vi "MatrixB.vi"(0 "No record Vg rate (V/min)":dbl=150.0, 3 "Time Stamp":timestamp, 4 "Voltage (sourse)":dbl, 6 "Play Button":bool, 8 "Custom Folder":string, 9 "Settings":T1={"Ring 3"=1, "Ring 2"=4, "Fixed Current mkA"=0.5, "If yes, the current is:"=enum."Radio Selection 1", "Ressitance measurements?"=TRUE, "Commute DC current?"=FALSE} {"Ring 3" items=["1 kOhm", "10 kOhm", "100 kOhm", "1 Mohm", "10 mOhm"]; "Ring 2" items=["1 kOhm", "10 kOhm", "100 kOhm", "1 Mohm", "10 MOhm"]}, 10 "Instruments":T2={"Oscillator"=TRUE, "Addr 1 lock-in"=TRUE, "Addr 1 lock-in oop"=TRUE, "Addr 2 lock-in"=TRUE, "Addr 2 lock-in oop"=TRUE, "Addr 3 lock-in"=FALSE, "Addr 3 lock-in oop"=FALSE, "Voltage (Vk1)"=TRUE, "Current (Ik1)"=TRUE, "Voltage (Vk2)"=FALSE, "Current (Ik2)"=FALSE, "Voltage (Vk3)"=FALSE, "Current (Ik3)"=FALSE, "Channel 1 (Vnano1)  "=FALSE, "Channel 2 (Vnano1b)"=FALSE, "Channel 1 (Vnano2)   "=FALSE, "Channel 2 (Vnano2b)"=FALSE, "Thermometer 1 (T1)"=TRUE, "Magnetic Field (B)"=TRUE, "Capacitance (C) and Loss (L)"=FALSE}, 11 "BCluster":T3={"B1 (T)"=-1.0, "B2 (T)"=1.0, "Sweep rate, T/min"=0.5, "Time btw \npoints, sec"=1.0, "No-record rate, T/min"=0.5, "Full sweep?"=FALSE, "Odd confgurations"=TRUE} {"No-record rate, T/min" min=0.0 max=1.0 step=0.01 format="%_4f"; "B2 (T)" min=-4.0 max=4.0 step=0.1 format="%.1f"; "Time btw \npoints, sec" format="%.2f"; "Sweep rate, T/min" min=0.0 max=1.0 step=0.01 format="%_4f"; "B1 (T)" min=-4.0 max=4.0 step=0.1 format="%.1f"}) -> ()   [LabVIEW 2017]
uses:
  <vilib>/Utility/file.llb/Read From Spreadsheet File (DBL).vi
panel:
  out "ArraySens 2":i8[](array[numeric])
  out "String":string
  out "Experiment ends at:":string
  out "Hours":dbl format="%.1f"
  out "Estimated time of experiment:":i16
  out "ArraySens":i8[](array[numeric])
  out "ArrayOsc":dbl[](array[numeric])
  out "# of configurations":i8
  out "Large Array":bool[][][](array[boolean])
  out "Contact configuration file (*.conf)":path
  # "hours"
  # "min.="
  # "Lock-in Amplifiers"
  # "Temperature"
  # "SourceMeters"
  # "Nanovoltmeters"
  # "Main"
  # "(not recommended, too slow)"
  # "Magnetic Field"
  # "Capacitance & Loss"
  # "(not recommended, too slow)"
  # ": B1 to B2, even: B2 to B1"
  # "(For hysteresis measurements)"
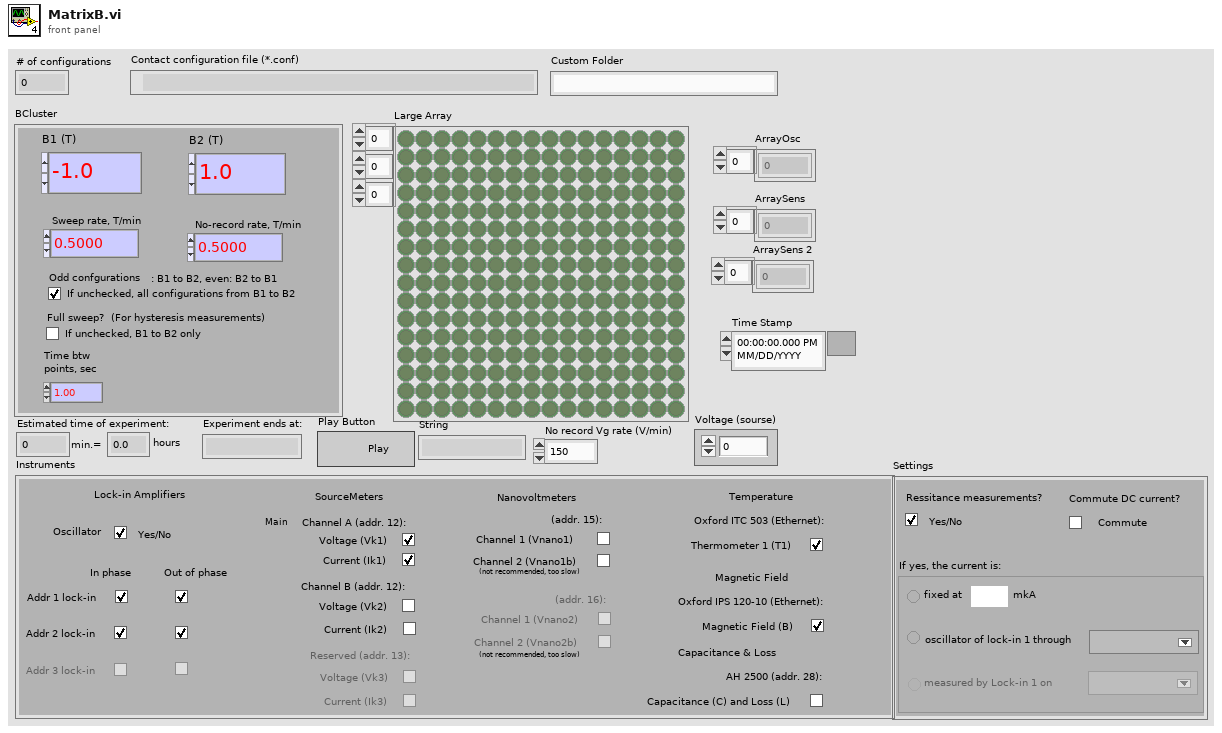
[diagram p1: front panel]
types:
  T1 = cluster{"Ring 3":u16, "Ring 2":u16, "Fixed Current mkA":dbl, "If yes, the current is:":enum32{"Radio Selection 1", "Radio Selection 2", "Radio Selection 3"}, "Ressitance measurements?":bool, "Commute DC current?":bool}
  T2 = cluster{"Oscillator":bool, "Addr 1 lock-in":bool, "Addr 1 lock-in oop":bool, "Addr 2 lock-in":bool, "Addr 2 lock-in oop":bool, "Addr 3 lock-in":bool, "Addr 3 lock-in oop":bool, "Voltage (Vk1)":bool, "Current (Ik1)":bool, "Voltage (Vk2)":bool, "Current (Ik2)":bool, "Voltage (Vk3)":bool, "Current (Ik3)":bool, "Channel 1 (Vnano1)  ":bool, "Channel 2 (Vnano1b)":bool, "Channel 1 (Vnano2)   ":bool, "Channel 2 (Vnano2b)":bool, "Thermometer 1 (T1)":bool, "Magnetic Field (B)":bool, "Capacitance (C) and Loss (L)":bool}
  T3 = cluster{"B1 (T)":dbl, "B2 (T)":dbl, "Sweep rate, T/min":dbl, "Time btw \npoints, sec":dbl, "No-record rate, T/min":dbl, "Full sweep?":bool, "Odd confgurations":bool}
  T4 = cluster{"B1 (T)":dbl, "Sweep rate, T/min":dbl, "Time btw \npoints, sec":dbl}
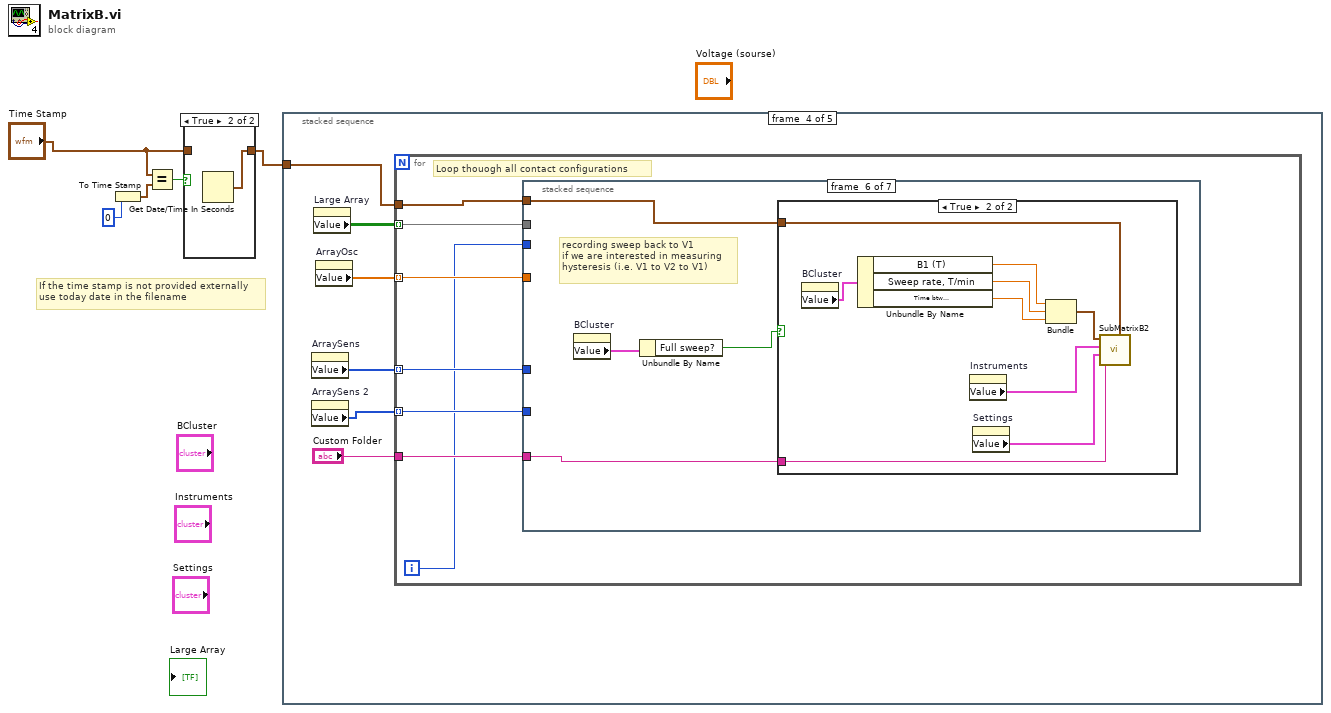
[diagram p0: block diagram]
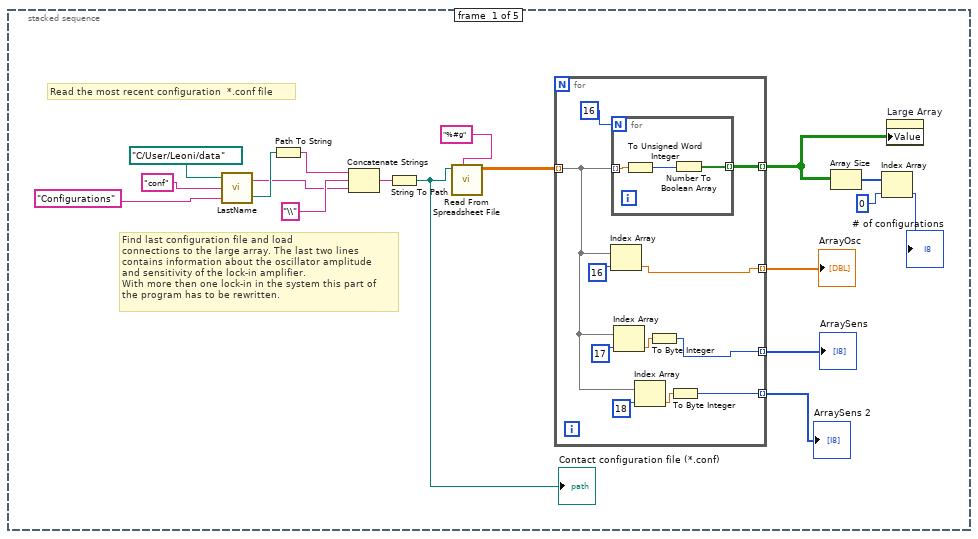
[diagram p3: hidden frame]
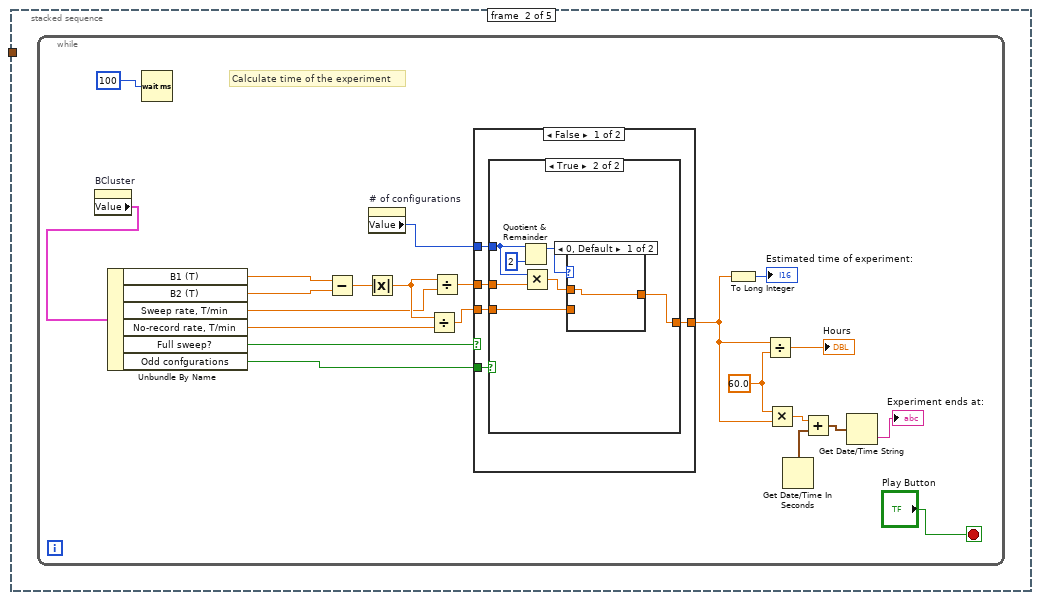
[diagram p4: hidden frame]
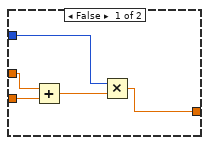
[diagram p5: hidden frame]
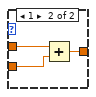
[diagram p6: hidden frame]
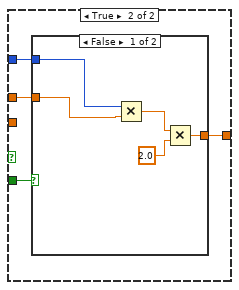
[diagram p7: hidden frame]
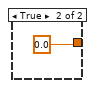
[diagram p8: hidden frame]
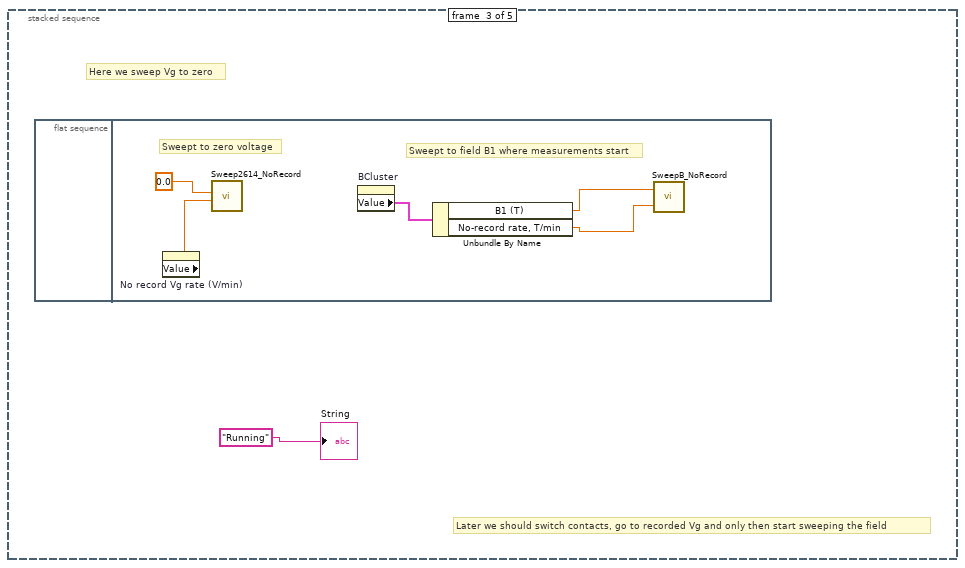
[diagram p9: hidden frame]
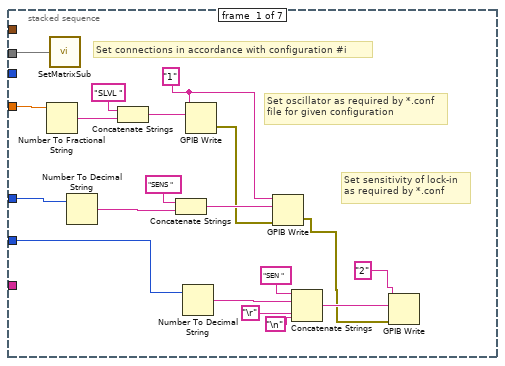
[diagram p10: hidden frame]
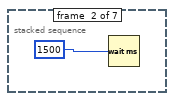
[diagram p11: hidden frame]
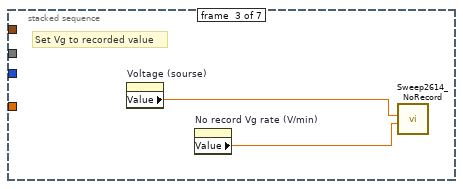
[diagram p12: hidden frame]
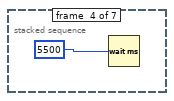
[diagram p13: hidden frame]
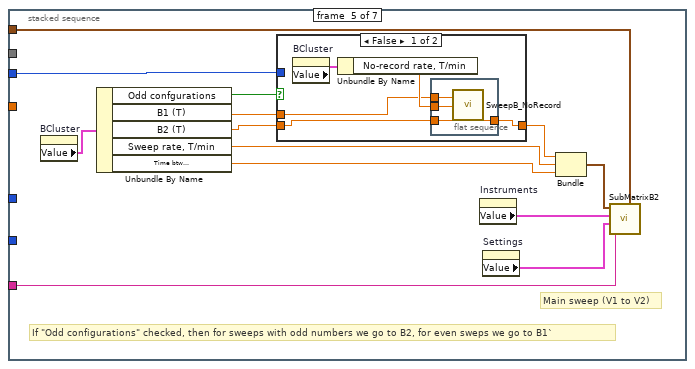
[diagram p14: hidden frame]
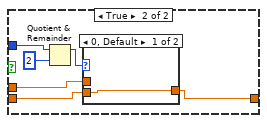
[diagram p15: hidden frame]
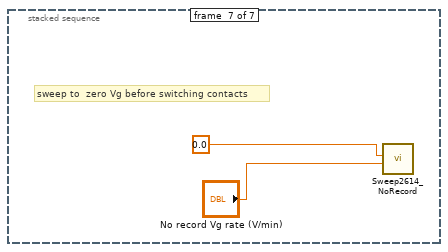
[diagram p18: hidden frame]
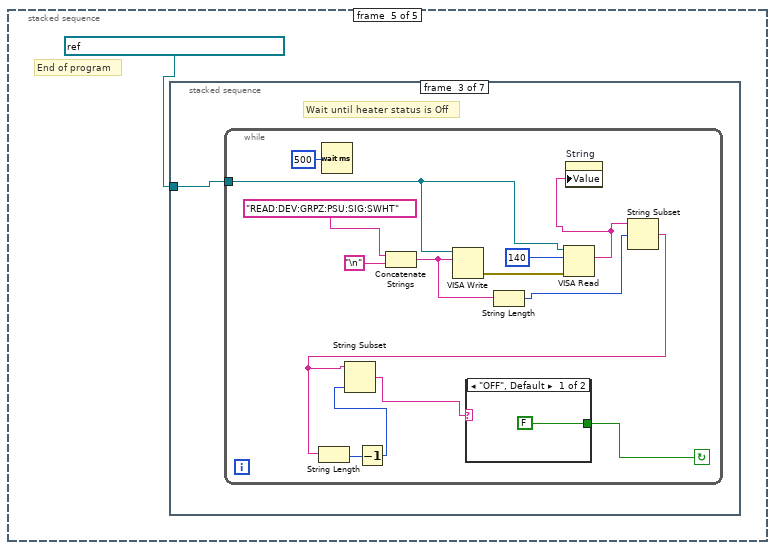
[diagram p19: hidden frame]
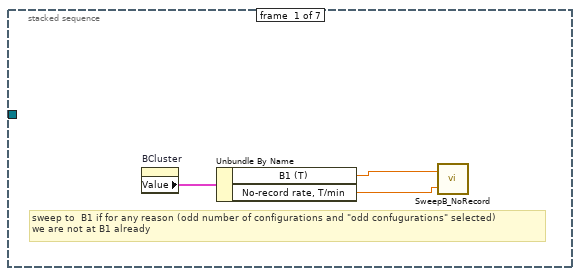
[diagram p20: hidden frame]
diagram:
  # "If the time stamp is not provided externally\nuse today date in the filename"
  n1 = To Time Stamp(1:0) -> (0:w4:timestamp)
  n2 = Equal?(x="Time Stamp", y=w4) -> (x = y?=w3:bool)
  n3 = case shown="True" w3 {
    tunnel: "Time Stamp" -> [w6 _]
    tunnel: [w6 w7] -> w1
    frame False {
    }
    frame True {
      n4 = Get Date/Time In Seconds() -> (seconds since 1Jan1904=w7:timestamp)
    }
  }
  n5 = stacked-sequence {
    tunnel: w1 -> [_ _ _ w100 _]
    frame #0 {
      # "Read the most recent configuration  *.conf file"
      # "Find last configuration file and load \nconnections to the large array. The last two lines \ncontains information about the oscillator amplitude\nand sensitivity of the lock-in amplifier.\nWith more then one lock-in in the system this part of \nthe program has to be rewritten."
      n6 = call "LastName.vi"("Custom Folder"="Configurations", "Extention"="conf", "User Data Folder"=path "C:/User/Leoni/data") -> ("created path"=w21:path, "String"=w20:string)
      n7 = Path To String(path=w21) -> (string=w25:string)
      n8 = Concatenate Strings(w25, "\\", w20) -> (w23:string)
      n9 = String To Path(string=w23) -> (path=w11:path)
      "Contact configuration file (*.conf)" <- w11
      n10 = call-poly <vilib>:"Read From Spreadsheet File.vi"("format (%.3f)"="%#g", "file path (dialog if empty)"=w11) -> ("all rows"=w16:dbl[][])  [unwired: 5 in, 4 out]
      n11 = for {
        tunnel: w16 -> [w27] mode=indexing
        tunnel: [w36] -> w13 mode=indexing
        tunnel: [w32] -> w10 mode=indexing
        tunnel: [w31] -> w9 mode=indexing
        tunnel: [w26] -> w8 mode=indexing
        n12 = Index Array(array=w27, index=16) -> (element=w32:dbl)
        n13 = for {
          N: 16 -> [_]
          tunnel: w27 -> [w39] mode=indexing
          tunnel: [w37] -> w36 mode=indexing
          n14 = To Unsigned Word Integer(number=w39) -> (unsigned 16bit integer=w38:u16)
          n15 = Number To Boolean Array(number=w38) -> (Boolean array=w37:bool[])
        }
        n16 = Index Array(array=w27, index=17) -> (element=w33:dbl)
        n17 = Index Array(array=w27, index=18) -> (element=w28:dbl)
        n18 = To Byte Integer(number=w33) -> (8bit integer=w31:i8)
        n19 = To Byte Integer(number=w28) -> (8bit integer=w26:i8)
      }
      "ArrayOsc" <- w10
      "ArraySens" <- w9
      "ArraySens 2" <- w8
      n20 = Array Size(array=w13) -> (size(s)=w15:i32[])
      n21 = Index Array(array=w15, index=0) -> (element=→"# of configurations":i32)
      n22 = property on="Large Array" class="Arr (strict)"("Value"=w13) -> ()  [unwired: 2 in, 2 out]
    }
    frame #1 {
      n23 = while {
        stop <- "Play Button" stop-if-true
        w47 = 60.0
        # "Calculate time of the experiment"
        n24 = property on="BCluster" class="Clust (strict)"() -> ("Value"=w59:T3)  [unwired: 2 in, 2 out]
        n25 = Unbundle By Name(w59) -> ("B1 (T)"=w58:dbl, "B2 (T)"=w57:dbl, "Sweep rate, T/min"=w54:dbl, "No-record rate, T/min"=w53:dbl, "Full sweep?"=w42:bool, "Odd confgurations"=w41:bool)
        n26 = Wait (ms)(milliseconds to wait=100) -> ()  [unwired: 1 out]
        n27 = Subtract(x=w58, y=w57) -> (x-y=w56:dbl)
        n28 = Absolute Value(x=w56) -> (abs(x)=w55:dbl)
        n29 = property on="# of configurations" class="DigNum (strict)"() -> ("Value"=w40:i8)  [unwired: 2 in, 2 out]
        n30 = Divide(x=w55, y=w53) -> (x/y=w43:dbl)
        n31 = Divide(x=w55, y=w54) -> (x/y=w44:dbl)
        n32 = case shown="False" w42 {
          tunnel: [w62 w86] -> w46
          tunnel: w44 -> [w66 w84]
          tunnel: w43 -> [w65 _]
          tunnel: w40 -> [w64 w83]
          tunnel: w41 -> [w63 w85]
          frame False {
            n33 = case shown="True" w63 {
              tunnel: w66 -> [w71 w75]
              tunnel: w65 -> [w70 w73]
              tunnel: w64 -> [w68 w76]
              tunnel: [w67 w72] -> w62
              frame False {
                n34 = Add(x=w71, y=w70) -> (x+y=w69:dbl)
                n35 = Multiply(x=w68, y=w69) -> (x*y=w67:dbl)
              }
              frame True {
                n36 = Quotient & Remainder(x=w76, y=2) -> (x-y*floor(x/y)=w77:i32)  [unwired: 1 out]
                n37 = Multiply(x=w76, y=w75) -> (x*y=w74:dbl)
                n38 = case shown="0, Default" w77 {
                  tunnel: w74 -> [w79 w82]
                  tunnel: w73 -> [_ w81]
                  tunnel: [w79 w80] -> w72
                  frame 0, Default {
                  }
                  frame 1 {
                    n39 = Add(x=w82, y=w81) -> (x+y=w80:dbl)
                  }
                }
              }
            }
          }
          frame True {
            n40 = case shown="False" w85 {
              tunnel: [w90 0.0] -> w86
              tunnel: w84 -> [w89 _]
              tunnel: w83 -> [w88 _]
              frame False {
                n41 = Multiply(x=w88, y=w89) -> (x*y=w87:dbl)
                n42 = Multiply(x=w87, y=2.0) -> (x*y=w90:dbl)
              }
              frame True {
              }
            }
          }
        }
        n43 = To Long Integer(number=w46) -> (32bit integer=→"Estimated time of experiment:":i32)
        n44 = Divide(x=w46, y=w47) -> (x/y=→"Hours":dbl)
        n45 = Multiply(x=w47, y=w46) -> (x*y=w45:dbl)
        n46 = Get Date/Time In Seconds() -> (seconds since 1Jan1904=w51:timestamp)
        n47 = Add(x=w45, y=w51) -> (x+y=w50:timestamp)
        n48 = Get Date/Time String(seconds (now)=w50) -> (time string=→"Experiment ends at:":string)  [unwired: 2 in, 1 out]
      }
    }
    frame #2 {
      # "Later we should switch contacts, go to recorded Vg and only then start sweeping the field"
      # "Here we sweep Vg to zero"
      n49 = flat-sequence {
        frame #0 {
        }
        frame #1 {
          # "Sweept to field B1 where measurements start"
          # "Sweept to zero voltage"
          n50 = property on="No record Vg rate (V/min)" class="DigNum (strict)"() -> ("Value"=w98:dbl)  [unwired: 2 in, 2 out]
          n51 = call "Sweep2614_NoRecord.vi"("Rate (V/min)"=w98, "Vfinal (V)"=0.0) -> ()  [unwired: 2 in, 1 out]
          n52 = property on="BCluster" class="Clust (strict)"() -> ("Value"=w96:T3)  [unwired: 2 in, 2 out]
          n53 = Unbundle By Name(w96) -> ("B1 (T)"=w94:dbl, "No-record rate, T/min"=w95:dbl)
          n54 = call "SweepB_NoRecord.vi"("Sweep Rate w/o recording (T/min)"=w95, "Target Field (T)"=w94) -> ()  [unwired: 2 in]
        }
      }
      "String" <- "Running"
    }
    frame #3 {
      n55 = property on="ArraySens" class="Arr (strict)"() -> ("Value"=w102:i8[])  [unwired: 2 in, 2 out]
      n56 = property on="ArraySens 2" class="Arr (strict)"() -> ("Value"=w99:i8[])  [unwired: 2 in, 2 out]
      n57 = property on="Large Array" class="Arr (strict)"() -> ("Value"=w104:bool[][][])  [unwired: 2 in, 2 out]
      n58 = property on="ArrayOsc" class="Arr (strict)"() -> ("Value"=w103:dbl[])  [unwired: 2 in, 2 out]
      n59 = for {
        tunnel: w104 -> [w111] mode=indexing
        tunnel: w103 -> [w110] mode=indexing
        tunnel: w102 -> [w109] mode=indexing
        tunnel: "Custom Folder" -> [w108]
        tunnel: w100 -> [w107]
        tunnel: w99 -> [w106] mode=indexing
        i -> [w105]
        # "Loop thouogh all contact configurations"
        n60 = stacked-sequence {
          tunnel: w111 -> [w130 _ _ _ _ _ _]
          tunnel: w110 -> [w126 _ _ _ _ _ _]
          tunnel: w109 -> [w121 _ _ _ _ _ _]
          tunnel: w108 -> [_ _ _ _ w147 w167 _]
          tunnel: w107 -> [_ _ _ _ w146 w166 _]
          tunnel: w106 -> [w113 _ _ _ _ _ _]
          tunnel: w105 -> [_ _ _ _ w136 _ _]
          frame #0 {
            w122 = "1"
            # "Set sensitivity of lock-in\nas required by *.conf"
            # "Set oscillator as required by *.conf\nfile for given configuration"
            # "Set connections in accordance with configuration #i"
            n61 = Number To Fractional String(number=w126) -> (F-format string=w129:string)  [unwired: 3 in]
            n62 = call "SetMatrixSub.vi"("Array"=w130) -> ()  [unwired: 1 in]
            n63 = Number To Decimal String(number=w121) -> (decimal integer string=w125:string)  [unwired: 1 in]
            n64 = Concatenate Strings("SLVL ", w129) -> (w128:string)
            n65 = Concatenate Strings("SENS ", w125) -> (w124:string)
            n66 = Number To Decimal String(number=w113) -> (decimal integer string=w119:string)  [unwired: 1 in]
            n67 = GPIB Write(0:w122, 1:w128) -> (6:w120:errorcluster)  [unwired: 3 in, 1 out]
            n68 = GPIB Write(0:w122, 1:w124, 3:w120) -> (6:w114:errorcluster)  [unwired: 2 in, 1 out]
            n69 = Concatenate Strings("SEN ", w119, "\r", "\n") -> (w118:string)
            n70 = GPIB Write(0:"2", 1:w118, 3:w114) -> ()  [unwired: 2 in, 2 out]
          }
          frame #1 {
            n71 = Wait (ms)(milliseconds to wait=1500) -> ()  [unwired: 1 out]
          }
          frame #2 {
            # "Set Vg to recorded value"
            n72 = property on="Voltage (sourse)" class="DigNum (strict)"() -> ("Value"=w133:dbl)  [unwired: 2 in, 2 out]
            n73 = property on="No record Vg rate (V/min)" class="DigNum (strict)"() -> ("Value"=w132:dbl)  [unwired: 2 in, 2 out]
            n74 = call "Sweep2614_NoRecord.vi"("Rate (V/min)"=w132, "Vfinal (V)"=w133) -> ()  [unwired: 2 in, 1 out]
          }
          frame #3 {
            n75 = Wait (ms)(milliseconds to wait=5500) -> ()  [unwired: 1 out]
          }
          frame #4 {
            # "If \"Odd configurations\" checked, then for sweeps with odd numbers we go to B2, for even sweps we go to B1`"
            # "Main sweep (V1 to V2)"
            n76 = property on="BCluster" class="Clust (strict)"() -> ("Value"=w145:T3)  [unwired: 2 in, 2 out]
            n77 = Unbundle By Name(w145) -> ("Odd confgurations"=w139:bool, "B1 (T)"=w135:dbl, "B2 (T)"=w138:dbl, "Sweep rate, T/min"=w144:dbl, "Time btw \npoints, sec"=w143:dbl)
            n78 = case shown="False" w139 {
              tunnel: w138 -> [w149 w158]
              tunnel: [w148 w157] -> w137
              tunnel: w136 -> [_ w159]
              tunnel: w135 -> [w150 w156]
              frame False {
                n79 = property on="BCluster" class="Clust (strict)"() -> ("Value"=w152:T3)  [unwired: 2 in, 2 out]
                n80 = Unbundle By Name(w152) -> ("No-record rate, T/min"=w151:dbl)
                n81 = flat-sequence {
                  tunnel: w151 -> [w155]
                  tunnel: w150 -> [w154]
                  tunnel: w149 -> [w153]
                  tunnel: [w153] -> w148
                  frame #0 {
                    n82 = call "SweepB_NoRecord.vi"("Sweep Rate w/o recording (T/min)"=w155, "Target Field (T)"=w154) -> ()  [unwired: 2 in]
                  }
                }
              }
              frame True {
                n83 = Quotient & Remainder(x=w159, y=2) -> (x-y*floor(x/y)=w160:i32)  [unwired: 1 out]
                n84 = case shown="0, Default" w160 {
                  tunnel: w158 -> [w162 _]
                  tunnel: [w162 w163] -> w157
                  tunnel: w156 -> [_ w163]
                  frame 0, Default {
                  }
                  frame 1 {
                  }
                }
              }
            }
            n85 = property on="Instruments" class="Clust (strict)"() -> ("Value"=w142:T2)  [unwired: 2 in, 2 out]
            n86 = property on="Settings" class="Clust (strict)"() -> ("Value"=w141:T1)  [unwired: 2 in, 2 out]
            n87 = Bundle("B1 (T)"=w137, "Sweep rate, T/min"=w144, "Time btw \npoints, sec"=w143) -> (w140:T4)  [unwired: 1 in]
            n88 = call "SubMatrixB2.vi"("BCluster"=w140, "Instruments"=w142, "Settings"=w141, "Custom Folder"=w147, "Time Stamp"=w146) -> ()  [unwired: 5 in]
          }
          frame #5 {
            # "recording sweep back to V1\nif we are interested in measuring \nhysteresis (i.e. V1 to V2 to V1)"
            n89 = property on="BCluster" class="Clust (strict)"() -> ("Value"=w165:T3)  [unwired: 2 in, 2 out]
            n90 = Unbundle By Name(w165) -> ("Full sweep?"=w164:bool)
            n91 = case shown="True" w164 {
              tunnel: w167 -> [_ w176]
              tunnel: w166 -> [_ w175]
              frame False {
              }
              frame True {
                n92 = property on="BCluster" class="Clust (strict)"() -> ("Value"=w174:T3)  [unwired: 2 in, 2 out]
                n93 = Unbundle By Name(w174) -> ("B1 (T)"=w173:dbl, "Sweep rate, T/min"=w172:dbl, "Time btw \npoints, sec"=w171:dbl)
                n94 = property on="Instruments" class="Clust (strict)"() -> ("Value"=w170:T2)  [unwired: 2 in, 2 out]
                n95 = property on="Settings" class="Clust (strict)"() -> ("Value"=w169:T1)  [unwired: 2 in, 2 out]
                n96 = Bundle("B1 (T)"=w173, "Sweep rate, T/min"=w172, "Time btw \npoints, sec"=w171) -> (w168:T4)  [unwired: 1 in]
                n97 = call "SubMatrixB2.vi"("BCluster"=w168, "Instruments"=w170, "Settings"=w169, "Custom Folder"=w176, "Time Stamp"=w175) -> ()  [unwired: 5 in]
              }
            }
          }
          frame #6 {
            # "sweep to  zero Vg before switching contacts"
            n98 = call "Sweep2614_NoRecord.vi"("Rate (V/min)"="No record Vg rate (V/min)", "Vfinal (V)"=0.0) -> ()  [unwired: 2 in, 1 out]
          }
        }
      }
    }
    frame #4 {
      # "End of program"
      n99 = stacked-sequence {
        tunnel: refnum<visa-resource-name> "TCPIP0::192.168.128.3::7020::SOCKET" ("VISA resource name") -> [_ w185 w190 _ w209 w215 _]
        frame #0 {
          # "sweep to  B1 if for any reason (odd number of configurations and \"odd confugurations\" selected)\nwe are not at B1 already"
          n100 = property on="BCluster" class="Clust (strict)"() -> ("Value"=w182:T3)  [unwired: 2 in, 2 out]
          n101 = Unbundle By Name(w182) -> ("B1 (T)"=w181:dbl, "No-record rate, T/min"=w180:dbl)
          n102 = call "SweepB_NoRecord.vi"("Sweep Rate w/o recording (T/min)"=w180, "Target Field (T)"=w181) -> ()  [unwired: 2 in]
        }
        frame #1 {
          # "Turn a switch heater OFF"
          n103 = Concatenate Strings("SET:DEV:GRPZ:PSU:SIG:SWHT:OFF" ("string"), "\n") -> (w186:string)
          n104 = VISA Write(VISA resource name=w185, write buffer=w186) -> (error out=w189:errorcluster)  [unwired: 1 in, 2 out]
          n105 = VISA Read(VISA resource name=w185, byte count=140, error in (no error)=w189) -> (read buffer=w183:string)  [unwired: 3 out]
          n106 = property on="String" class="Str"("Value"=w183) -> ()  [unwired: 2 in, 2 out]
        }
        frame #2 {
          # "Wait until heater status is Off"
          n107 = while {
            tunnel: w190 -> [w201]
            stop <- w193 continue-if-true
            n108 = Wait (ms)(milliseconds to wait=500) -> ()  [unwired: 1 out]
            n109 = Concatenate Strings("READ:DEV:GRPZ:PSU:SIG:SWHT" ("string"), "\n") -> (w200:string)
            n110 = VISA Write(VISA resource name=w201, write buffer=w200) -> (error out=w204:errorcluster)  [unwired: 1 in, 2 out]
            n111 = String Length(string=w200) -> (length=w199:i32)
            n112 = VISA Read(VISA resource name=w201, byte count=140, error in (no error)=w204) -> (read buffer=w191:string)  [unwired: 3 out]
            n113 = property on="String" class="Str"("Value"=w191) -> ()  [unwired: 2 in, 2 out]
            n114 = String Subset(string=w191, offset (0)=w199) -> (substring=w192:string)  [unwired: 1 in]
            n115 = String Length(string=w192) -> (length=w196:i32)
            n116 = Decrement(x=w196) -> (x-1=w195:i32)
            n117 = String Subset(string=w192, length (rest)=w195) -> (substring=w194:string)  [unwired: 1 in]
            n118 = case shown="\"OFF\", Default" w194 {
              tunnel: [FALSE TRUE] -> w193
              frame "OFF", Default {
              }
              frame "ON" {
              }
            }
          }
        }
        frame #3 {
          n119 = Wait (ms)(milliseconds to wait=15000) -> ()  [unwired: 1 out]
        }
        frame #4 {
          # "Ramp the magnet to zero (persistant mode)"
          n120 = Concatenate Strings("SET:DEV:GRPZ:PSU:ACTN:RTOZ" ("string"), "\n") -> (w211:string)
          n121 = VISA Write(VISA resource name=w209, write buffer=w211) -> (error out=w214:errorcluster)  [unwired: 1 in, 2 out]
          n122 = VISA Read(VISA resource name=w209, byte count=140, error in (no error)=w214) -> (read buffer=w208:string)  [unwired: 3 out]
          n123 = property on="String" class="Str"("Value"=w208) -> ()  [unwired: 2 in, 2 out]
        }
        frame #5 {
          # "Step 4. Wait until the magnet reached HOLD state."
          n124 = while {
            tunnel: w215 -> [w225]
            stop <- w218 stop-if-true
            n125 = Wait (ms)(milliseconds to wait=500) -> ()  [unwired: 1 out]
            n126 = Concatenate Strings("READ:DEV:GRPZ:PSU:ACTN" ("string"), "\n") -> (w222:string)
            n127 = VISA Write(VISA resource name=w225, write buffer=w222) -> (error out=w228:errorcluster)  [unwired: 1 in, 2 out]
            n128 = String Length(string=w222) -> (length=w221:i32)
            n129 = VISA Read(VISA resource name=w225, byte count=140, error in (no error)=w228) -> (read buffer=w216:string)  [unwired: 3 out]
            n130 = property on="String" class="Str"("Value"=w216) -> ()  [unwired: 2 in, 2 out]
            n131 = String Subset(string=w216, offset (0)=w221, length (rest)=4) -> (substring=w220:string)
            n132 = Equal?(x=w220, y="HOLD") -> (x = y?=w218:bool)
          }
        }
        frame #6 {
          n133 = property on="String" class="Str"("Value"="") -> ()  [unwired: 2 in, 2 out]
        }
      }
    }
  }
